vi "LowIF_audiojack.vi"() -> ()   [LabVIEW 2014]
doc: "This example demonstrates how to use the Short-time Fourier Transform (STFT Spectrograms) VI to analyze the Time-Frequency spectrogram."
uses:
  <vilib>/sound2/lvsound2.llb/Sampling Mode.ctl
  <vilib>/Analysis/2dsp.llb/Complex FFT.vi
  <vilib>/sound2/lvsound2.llb/Sound Input Read (DBL).vi
  <vilib>/Analysis/baseanly.llb/Mean (CDB).vi
  <vilib>/Analysis/NI_AALPro.lvlib
  <vilib>/Analysis/NI_AALBase.lvlib
panel:
  in  "scale to beats per min?":bool
  in  "Minimun dB":dbl=-15.0 max=0.0
  in  "dB scale?":bool
  in  "Frequency Range":dbl(slide)=3.2 caption="Frequency range" min=1.0 step=0.1 scale=0.0..160.0
  in  "negative frequency?":bool=TRUE
  out "Frequency":dbl[](graph) caption="I/Q Signal"
  in  "bits per sample":i32=16
  in  "number of channels":i32=2
  in  "sample rate (S/s)":dbl=320.0
  in  "data length":i32=6400
  out "I/Q Signal":dynamicdata(graph)
  in  "number of samples/ch":i32=32
  in  "device ID":u32
  in  "Stop":bool
  # "Low-IF interferometry radar data processing"
  # "Version: 2\nZhengyu Peng\nC. Li Lab\nTexas Tech University\nSep. 2015"
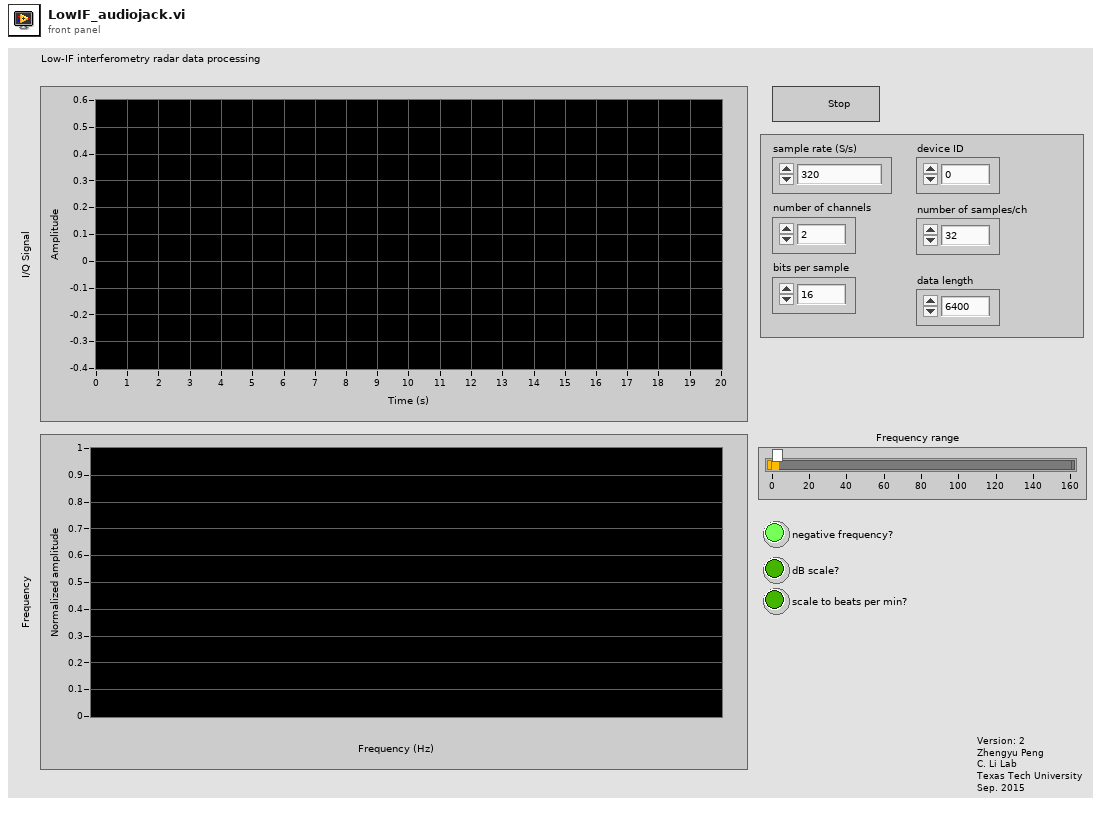
[diagram p1: front panel]
types:
  T1 = typedef "Sampling Mode.ctl" = i32
  T2 = cluster{"sample rate (S/s)":dbl, "number of channels":i32, "bits per sample ":i32}
  T3 = typedef "Sound Input Task ID.ctl" = u32
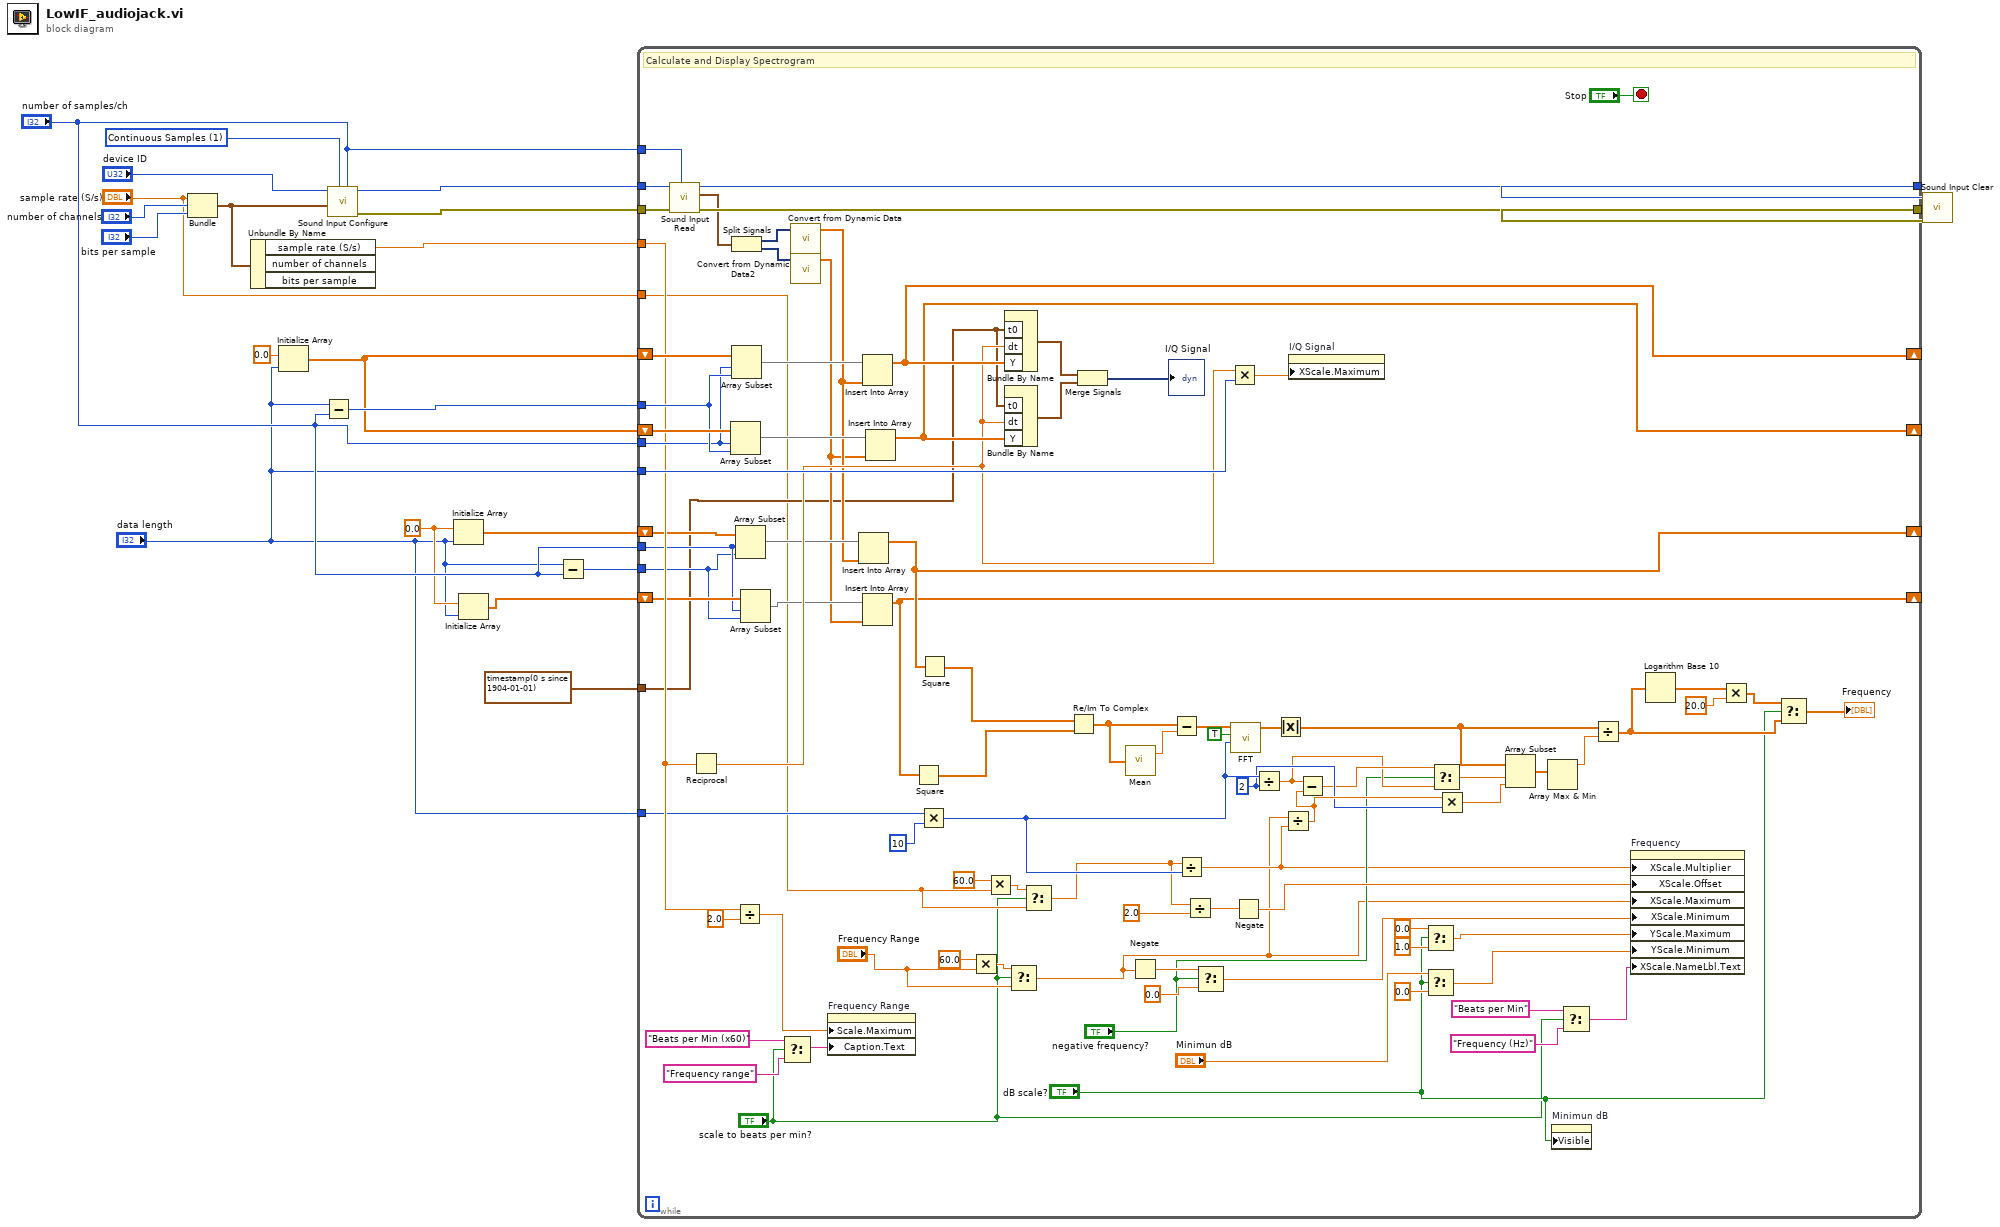
[diagram p0: block diagram]
diagram:
  w3 = T1 1 items=["Finite Samples", "Continuous Samples"] ("sample mode")
  w6 = 0.0 ("element")
  n1 = Bundle("sample rate (S/s)"="sample rate (S/s)", "number of channels"="number of channels", "bits per sample"="bits per sample") -> (w10:T2)  [unwired: 1 in]
  n2 = Unbundle By Name(w10) -> ("sample rate (S/s)"=w13:dbl)  [unwired: 2 out]
  n3 = Initialize Array(0.0 ("element"), "data length") -> (w14:dbl[])
  n4 = Subtract(x="data length", y="number of samples/ch") -> (x-y=w15:i32)
  n5 = call <vilib>:"Sound Input Configure.vi"("number of samples/ch"="number of samples/ch", "sample mode"=w3, "sound format"=w10, "device ID"="device ID") -> ("error out"=w19:errorcluster, "task ID"=w20:T3)  [unwired: 6 in]
  n6 = Initialize Array(w6, "data length") -> (w9:dbl[])
  n7 = Initialize Array(w6, "data length") -> (w5:dbl[])
  n8 = Subtract(x="data length", y="number of samples/ch") -> (x-y=w8:i32)
  n9 = while {
    tunnel: w20 -> [w111]
    tunnel: "number of samples/ch" -> [w110]
    tunnel: w19 -> [w109]
    tunnel: [w108] -> w18
    tunnel: [w107] -> w17
    shift-right: [w91] -> _
    shift-left: w14 -> [w103]
    tunnel: w15 -> [w100]
    shift-right: [w90] -> _
    shift-left: w14 -> [w101]
    tunnel: "number of samples/ch" -> [w97]
    tunnel: w13 -> [w93]
    tunnel: "data length" -> [w95]
    tunnel: "data length" -> [w73]
    tunnel: "sample rate (S/s)" -> [w31]
    shift-right: [w71] -> _
    shift-left: w9 -> [w81]
    tunnel: w8 -> [w76]
    tunnel: "number of samples/ch" -> [w77]
    shift-right: [w70] -> _
    shift-left: w5 -> [w78]
    tunnel: timestamp(0 s since 1904-01-01) ("t0") -> [w66]
    stop <- "Stop" stop-if-true
    w55 = 2 ("y")
    # "Calculate and Display Spectrogram"
    n10 = call-poly <vilib>:"Sound Input Read.vi"("number of samples/ch"=w110, "error in (no error)"=w109, "task ID"=w111) -> ("error out"=w107:errorcluster, "data"=w104:waveform(dbl)[], "task ID out"=w108:T3)  [unwired: 6 in]
    n11 = Reciprocal(x=w93) -> (1/x=w85:dbl)
    n12 = Array Subset(array=w101, index=w97, length=w100) -> (w99:dbl[])
    n13 = Split Signals(w104) -> (w106:dynamicdata, w105:dynamicdata)  [unwired: 2 out]
    n14 = Array Subset(array=w103, index=w97, length=w100) -> (w102:dbl[])
    n15 = Divide(x=w93, y=2.0) -> (x/y=w65:dbl)
    n16 = Array Subset(array=w81, index=w77, length=w76) -> (w80:dbl[])
    n17 = Array Subset(array=w78, index=w77, length=w76) -> (w75:dbl[])
    n18 = Select(t="Beats per Min (x60)" ("X Scale.Name Label.Text"), s="scale to beats per min?", f="Frequency range" ("X Scale.Name Label.Text")) -> (s? t:f=w23:string)
    n19 = call "Convert from Dynamic Data"("Dynamic Data Type"=w106) -> ("Array"=w79:dbl[])  [unwired: 3 out]
    n20 = call "Convert from Dynamic Data2"("Dynamic Data Type"=w105) -> ("Array"=w74:dbl[])  [unwired: 3 out]
    n21 = property on="Frequency Range" class="Slide (strict)"("Scale.Maximum"=w65, "Caption.Text"=w23) -> ()  [unwired: 2 in, 2 out]
    n22 = Insert Into Array(array=w80, new element=w79) -> (w71:dbl[])  [unwired: 1 in]
    n23 = Insert Into Array(array=w102, new element=w79) -> (w91:dbl[])  [unwired: 1 in]
    n24 = Insert Into Array(array=w75, new element=w74) -> (w70:dbl[])  [unwired: 1 in]
    n25 = Insert Into Array(array=w99, new element=w74) -> (w90:dbl[])  [unwired: 1 in]
    n26 = Square(x=w70) -> (x^2=w68:dbl[])
    n27 = Multiply(x=w73, y=10) -> (x*y=w58:i32)
    n28 = Square(x=w71) -> (x^2=w69:dbl[])
    n29 = Multiply(x=60.0, y="Frequency Range") -> (x*y=w29:dbl)
    n30 = Multiply(x=60.0, y=w31) -> (x*y=w34:dbl)
    n31 = Bundle By Name("t0"=w66, "dt"=w85, "Y"=w91) -> (w98:waveform(dbl))  [unwired: 1 out]
    n32 = Bundle By Name("t0"=w66, "dt"=w85, "Y"=w90) -> (w96:waveform(dbl))  [unwired: 1 out]
    n33 = Select(t=w29, s="scale to beats per min?", f="Frequency Range") -> (s? t:f=w28:dbl)
    n34 = Select(t=w34, s="scale to beats per min?", f=w31) -> (s? t:f=w32:dbl)
    n35 = Re/Im To Complex(1:w68, 2:w69) -> (0:w89:cdb[])
    n36 = Merge Signals(w98, w96) -> (→"I/Q Signal":dynamicdata)
    n37 = call-poly <vilib>:"Mean.vi"("X"=w89) -> ("mean"=w88:cdb)  [unwired: 1 out]
    n38 = Negate(x=w28) -> (-x=w62:dbl)
    n39 = Subtract(x=w89, y=w88) -> (x-y=w67:cdb[])
    n40 = Divide(x=w32, y=w58) -> (x/y=w33:dbl)
    n41 = Divide(x=w32, y=2.0) -> (x/y=w83:dbl)
    n42 = Select(t=w62, s="negative frequency?", f=0.0) -> (s? t:f=w64:dbl)
    n43 = Multiply(x=w85, y=w95) -> (x*y=w94:dbl)
    n44 = call-poly <vilib>:"FFT.vi"("FFT size"=w58, "shift?"=TRUE, "X"=w67) -> ("FFT {X}"=w86:cdb[])  [unwired: 7 in, 1 out]
    n45 = Negate(x=w83) -> (-x=w82:dbl)
    n46 = Divide(x=w58, y=w55) -> (x/y=w52:dbl)
    n47 = Absolute Value(x=w86) -> (abs(x)=w61:dbl[])
    n48 = Divide(x=w28, y=w33) -> (x/y=w56:dbl)
    n49 = property on="I/Q Signal" class="WFGraph (strict)"("XScale.Maximum"=w94) -> ()  [unwired: 2 in, 2 out]
    n50 = Subtract(x=w52, y=w56) -> (x-y=w53:dbl)
    n51 = Select(t=0.0, s="dB scale?", f=1.0) -> (s? t:f=w42:dbl)
    n52 = Select(t="Minimun dB", s="dB scale?", f=0.0) -> (s? t:f=w46:dbl)
    n53 = Select(t=w53, s="negative frequency?", f=w52) -> (s? t:f=w54:dbl)
    n54 = Multiply(x=w56, y=w55) -> (x*y=w57:dbl)
    n55 = Array Subset(array=w61, index=w54, length=w57) -> (w60:dbl[])
    n56 = Array Max & Min(array=w60) -> (max value=w59:dbl)  [unwired: 3 out]
    n57 = property on="Minimun dB" class="DigNum (strict)"("Visible"="dB scale?") -> ()  [unwired: 2 in, 2 out]
    n58 = Select(t="Beats per Min" ("X Scale.Name Label.Text"), s="scale to beats per min?", f="Frequency (Hz)" ("X Scale.Name Label.Text")) -> (s? t:f=w37:string)
    n59 = Divide(x=w61, y=w59) -> (x/y=w40:dbl[])
    n60 = property on="Frequency" class="WFGraph (strict)"("XScale.Multiplier"=w33, "XScale.Offset"=w82, "XScale.Maximum"=w28, "XScale.Minimum"=w64, "YScale.Maximum"=w42, "YScale.Minimum"=w46, "XScale.NameLbl.Text"=w37) -> ()  [unwired: 2 in, 2 out]
    n61 = Logarithm Base 10(1:w40) -> (0:w50:dbl[])
    n62 = Multiply(x=w50, y=20.0) -> (x*y=w48:dbl[])
    n63 = Select(t=w48, s="dB scale?", f=w40) -> (s? t:f=→"Frequency":dbl[])
  }
  n64 = call <vilib>:"Sound Input Clear.vi"("error in (no error)"=w17, "task ID"=w18) -> ()  [unwired: 9 in, 1 out]
